vi "Calc_Allan-Variance.VI"(2 "Input Array":dbl[](array[numeric]) format="%.2f") -> (0 "AllanVariance":dbl[](array[numeric]))   [LabVIEW 2023]
uses:
  <vilib>/Analysis/baseanly.llb/Mean (DBL).vi
  <vilib>/Analysis/NI_AALBase.lvlib
panel:
  out "[y_mean(k+1) - y_mean(k)]**2":dbl[](array[numeric]) format="%.3f"
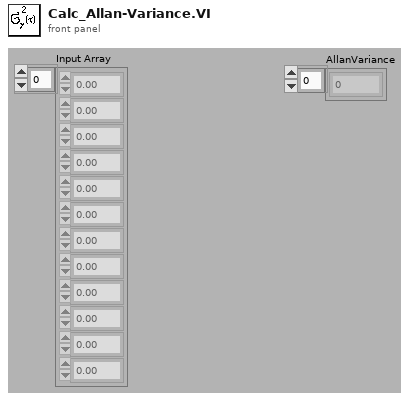
[diagram p1: front panel]
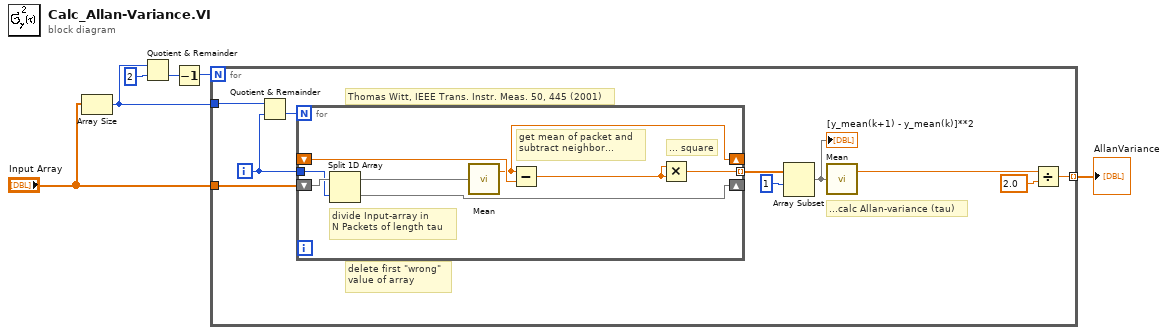
[diagram p0: block diagram]
diagram:
  n1 = Array Size(array="Input Array") -> (size(s)=w2:i32)
  n2 = Quotient & Remainder(x=w2, y=2) -> (floor(x/y)=w3:i32)  [unwired: 1 out]
  n3 = Decrement(x=w3) -> (x-1=w1:i32)
  n4 = for {
    N: w1 -> [_]
    tunnel: w2 -> [w16]
    tunnel: "Input Array" -> [w15]
    tunnel: [w8] -> w5 mode=indexing
    i -> [w7]
    # "Thomas Witt, IEEE Trans. Instr. Meas. 50, 445 (2001)"
    # "delete first \"wrong\"\nvalue of array"
    # "...calc Allan-variance (tau)"
    n5 = Quotient & Remainder(x=w16, y=w7) -> (floor(x/y)=w14:i32)  [unwired: 1 out]
    n6 = for {
      N: w14 -> [_]
      shift-right: [w23] -> _
      shift-left: w15 -> [w24]
      tunnel: w7 -> [w17]
      shift-right: [w20] -> _
      shift-left: _ -> [w21]
      tunnel: [w18] -> w11 mode=indexing
      # "... square"
      # "get mean of packet and\nsubtract neighbor..."
      # "divide Input-array in\nN Packets of length tau"
      n7 = Split 1D Array(array=w24, index=w17) -> (first subarray=w22:dbl[], second subarray=w23:dbl[])
      n8 = call-poly <vilib>:"Mean.vi"("X"=w22) -> ("mean"=w20:dbl)  [unwired: 1 out]
      n9 = Subtract(x=w20, y=w21) -> (x-y=w19:dbl)
      n10 = Multiply(x=w19, y=w19) -> (x*y=w18:dbl)
    }
    n11 = Array Subset(array=w11, index=1 ("mean")) -> (w9:dbl[])  [unwired: 1 in]
    "[y_mean(k+1) - y_mean(k)]**2" <- w9
    n12 = call-poly <vilib>:"Mean.vi"("X"=w9) -> ("mean"=w13:dbl)  [unwired: 1 out]
    n13 = Divide(x=w13, y=2.0) -> (x/y=w8:dbl)
  }
  "AllanVariance" <- w5
